vi "RichTextDemo.vi"() -> ()   [LabVIEW 2012]
uses:
  RichTextClass/Basic RichText Property.ctl
  RichTextClass/RichText.lvclass
  System.Windows.Forms
panel:
  in  "停止":bool
  in  "RichTextBox":refnum<k24>(container)
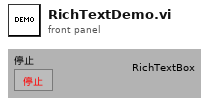
[diagram p1: front panel]
types:
  T1 = typedef "RichText.lvclass/Basic RichText Property.ctl" = cluster{"familyName":string, "emSize":sgl, "newStyle":i32, "color":i32, "BackColor":i32}
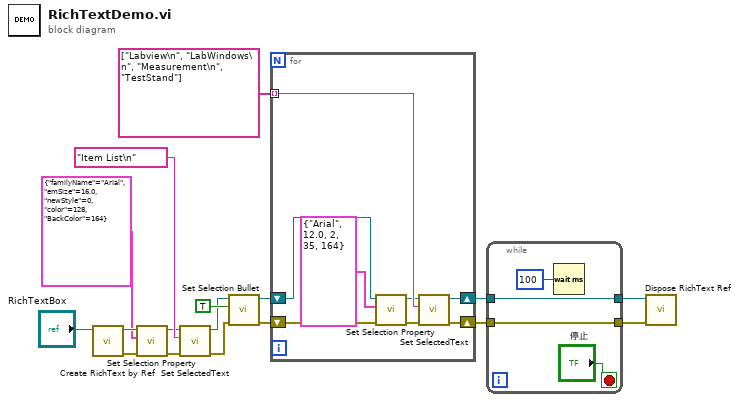
[diagram p0: block diagram]
diagram:
  n1 = call "Create RichText by Ref.vi"("RichTextBox"="RichTextBox") -> ("error out"=w8:errorcluster, "RichText 输出"=w9:refnum<class "RichText.lvclass">)  [unwired: 9 in]
  n2 = call "Set Selection Property.vi"("error in (no error)"=w8, "RichText Prop"=T1 {"familyName"="Arial", "emSize"=16.0, "newStyle"=0, "color"=128, "BackColor"=164}, "RichText 输入"=w9) -> ("error out"=w5:errorcluster, "RichText 输出"=w6:refnum<class "RichText.lvclass">)  [unwired: 7 in]
  n3 = call "Set SelectedText.vi"("error in (no error)"=w5, "SelectedText"="Item List\n", "RichText 输入"=w6) -> ("error out"=w3:errorcluster, "RichText 输出"=w4:refnum<class "RichText.lvclass">)  [unwired: 7 in]
  n4 = call "Set Selection Bullet.vi"("error in (no error)"=w3, "SelectionBullet"=TRUE, "RichText 输入"=w4) -> ("error out"=w12:errorcluster, "RichText 输出"=w13:refnum<class "RichText.lvclass">)  [unwired: 7 in]
  n5 = for {
    shift-right: [w25] -> w15
    shift-left: w13 -> [w22]
    shift-right: [w24] -> w14
    shift-left: w12 -> [w21]
    tunnel: string[] ["Labview\n", "LabWindows\n", "Measurement\n", "TestStand"] -> [w23] mode=indexing
    n6 = call "Set Selection Property.vi"("error in (no error)"=w21, "RichText Prop"=T1 {"familyName"="Arial", "emSize"=12.0, "newStyle"=2, "color"=35, "BackColor"=164}, "RichText 输入"=w22) -> ("error out"=w20:errorcluster, "RichText 输出"=w19:refnum<class "RichText.lvclass">)  [unwired: 7 in]
    n7 = call "Set SelectedText.vi"("error in (no error)"=w20, "SelectedText"=w23, "RichText 输入"=w19) -> ("error out"=w24:errorcluster, "RichText 输出"=w25:refnum<class "RichText.lvclass">)  [unwired: 7 in]
  }
  n8 = while {
    tunnel: [w26] -> w1
    tunnel: [w27] -> w2
    tunnel: w15 -> [w27]
    tunnel: w14 -> [w26]
    stop <- "停止" stop-if-true
    n9 = Wait (ms)(milliseconds to wait=u32 100 ("等待时间（毫秒）")) -> ()  [unwired: 1 out]
  }
  n10 = call "Dispose RichText Ref.vi"("error in (no error)"=w1, "RichText 输入"=w2) -> ()  [unwired: 8 in, 2 out]
